vi "Check Protection.vi"(8 "error in (no error)":errorcluster, 10 "String in":string, 11 "CRC-32 in":refnum<class "CRC-32.lvclass">) -> (0 "error out":errorcluster, 1 "Protection Error":errorcluster, 2 "String out":string, 3 "CRC-32 out":refnum<class "CRC-32.lvclass">)   [LabVIEW 2023, in "Protections.lvlib" / "CRC-32.lvclass"]
uses:
  CRC-32.lvclass
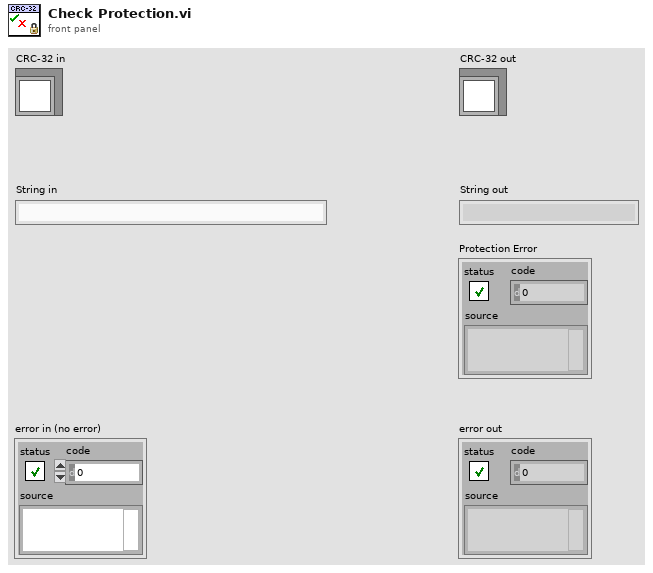
[diagram p1: front panel]
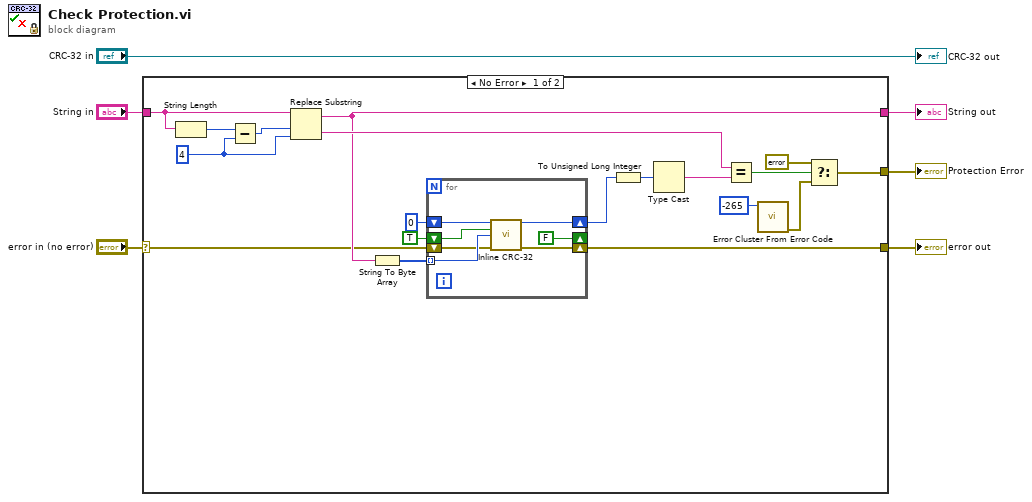
[diagram p0: block diagram]
diagram:
  n1 = case shown="No Error" "error in (no error)" {
    selector: "error in (no error)" -> [w9 w33]
    tunnel: "String in" -> [w16 w34]
    tunnel: [w14 _] -> w2
    tunnel: [w15 w34] -> w3
    tunnel: [w8 w33] -> w1
    frame No Error {
      w23 = 4
      n2 = String Length(string=w16) -> (length=w25:i32)
      n3 = Subtract(x=w25, y=w23) -> (x-y=w24:i32)
      n4 = Replace Substring(2:w23, 3:w24, 5:w16) -> (0:w21:string, 1:w15:string)  [unwired: 1 in]
      n5 = String To Byte Array(string=w15) -> (unsigned byte array=w10:u8[])
      n6 = for {
        shift-right: [w31] -> w7
        shift-left: u32 0 ("CRC") -> [w32]
        tunnel: w10 -> [w30] mode=indexing
        shift-right: [w28] -> w8
        shift-left: w9 -> [w29]
        shift-right: [FALSE] -> _
        shift-left: TRUE -> [w27]
        n7 = call "Inline CRC-32.vi"("CRC In"=w32, "Reset"=w27, "Data"=w30, "error in (no error)"=w29) -> ("CRC"=w31:u32, "error out"=w28:errorcluster)  [unwired: 10 in]
      }
      n8 = To Unsigned Long Integer(number=w7) -> (unsigned 32bit integer=w13:u32)
      n9 = Type Cast(x=w13) -> (*(type *) &x=w22:string)  [unwired: 1 in]
      n10 = Equal?(x=w21, y=w22) -> (x = y?=w20:bool)
      n11 = call <vilib>:"Error Cluster From Error Code.vi"("error code (0)"=-265) -> ("error out"=w18:errorcluster)  [unwired: 8 in]
      n12 = Select(t=errorcluster {"status"=FALSE, "code"=0, "source"=""} ("error in (no error)"), s=w20, f=w18) -> (s? t:f=w14:errorcluster)
    }
    frame Error {
    }
  }
  "error out" <- w1
  "String out" <- w3
  "Protection Error" <- w2
  "CRC-32 out" <- "CRC-32 in"
